vi "3D Surface graph.vi"() -> (0 "Longitude out":dbl format="%.2f", 1 "Latitude out":dbl format="%.2f", 2 "3D graph out":refnum<k7>)   [LabVIEW 2013]
uses:
  <vilib>/Platform/NI_3dgraph.lvlib
panel:
  in  "3D Surface":refnum<k7>(container)
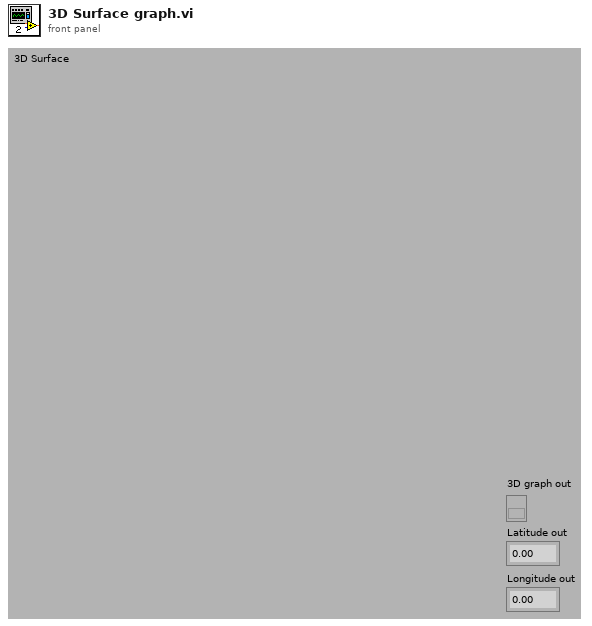
[diagram p1: front panel]
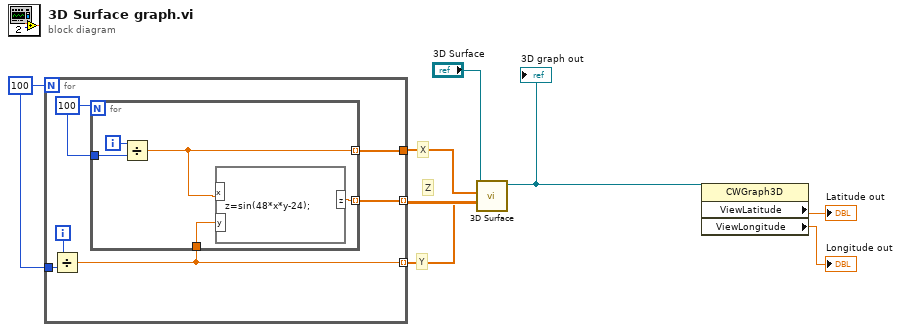
[diagram p0: block diagram]
diagram:
  w7 = 100
  # "Z"
  # "X"
  # "Y"
  n1 = for {
    N: w7 -> [_]
    tunnel: w7 -> [w12]
    tunnel: [w10] -> w4 mode=indexing
    tunnel: [w11] -> w5
    tunnel: [w9] -> w6 mode=indexing
    i -> [w13]
    w14 = 100
    n2 = Divide(x=w13, y=w12) -> (x/y=w10:dbl)
    n3 = for {
      N: w14 -> [_]
      tunnel: w14 -> [w18]
      tunnel: [w17] -> w11 mode=indexing
      tunnel: w10 -> [w16]
      tunnel: [w15] -> w9 mode=indexing
      i -> [w19]
      n4 = Divide(x=w19, y=w18) -> (x/y=w17:dbl)
      n5 = formula code="z=sin(48*x*y-24);"("y"=w16, "x"=w17) -> ("z"=w15:dbl)
    }
  }
  n6 = call <vilib>:"3D Surface.vi"("z matrix"=w6, "y vector"=w4, "x vector"=w5, "3D graph"="3D Surface") -> ("3D graph out"=w3:refnum<k7>)  [unwired: 1 in, 6 out]
  "3D graph out" <- w3
  n7 = property class="CWGraph3D"(reference=w3) -> ("ViewLatitude"=→"Latitude out":dbl, "ViewLongitude"=→"Longitude out":dbl)  [unwired: 1 in, 2 out]
